vi "BalancePressure4.vi"(0 "FirgelliError":errorcluster, 1 "length":dbl=50.0 caption="Actuator Length (mm)", 2 "DesiredPressure":dbl=-0.08 min=-1.0 max=0.0 step=0.001, 3 "Position (mm)":dbl(slide)=25.0 min=0.0 max=50.0 step=0.2 scale=0.0..50.0 scale format="%.2f", 4 "ArduinoHandle":T2={"VISA resource"="", "Board Type"=enum."Uno", "Connection Type"=enum."USB / Serial", "Bytes Per Packet (15)"=15}, 5 "CurrentPressure":dbl, 6 "WRITE_HANDLE":u32 format="%04x", 7 "PressureOffset":dbl, 8 "READ_HANDLE":u32 format="%04x", 9 "Control Values":T1, 10 "Transducer (psi)":dbl(ring)=1.0 items=["+/- .18 psi"=1.0, "+/- .36 psi"=2.0, "+/- 1.08 psi"=3.0], 11 "Syringe (mL)":dbl(ring)=1.0 items=[".5 mL"=2.0, "1 mL"=1.0, "3 mL"=3.0]) -> (14 "FirgelliError Out":errorcluster, 15 "Control Values Out":T1, 16 "UpdateChart?":bool, 17 "Position (mm) Out":dbl(slide)=25.0 min=0.0 max=50.0 step=0.2 scale=0.0..50.0 scale format="%.2f", 18 "ArduinoError Out":errorcluster, 19 "Pressure (psi)":dbl)   [LabVIEW 2011]
uses:
  <vilib>/LabVIEW Interface for Arduino/Type Defs/Arduino Resource.ctl
  <vilib>/LabVIEW Interface for Arduino/Type Defs/Board Type.ctl
  orders/Firgelli motor/LAC_Software_V2/Firgelli Labview Example/Firgelli_LAC_LabVIEWsourceVer8_2/typeDefs/controlValues.ctl
  <vilib>/LabVIEW Interface for Arduino/LabVIEW Interface for Arduino.lvlib
panel:
  in  "Accuracy":dbl
  in  "P":dbl=4.0
  in  "stop 2":bool
  in  "stop":bool
  in  "D":dbl
  in  "I":dbl
  out "LastError":dbl
  out "Error":dbl
  out "LastPressure":dbl
  in  "ArduinoError":errorcluster
  in  "Analog Input Pin (0)":u8=1
  in  "Valve I/O Pin":u8=2
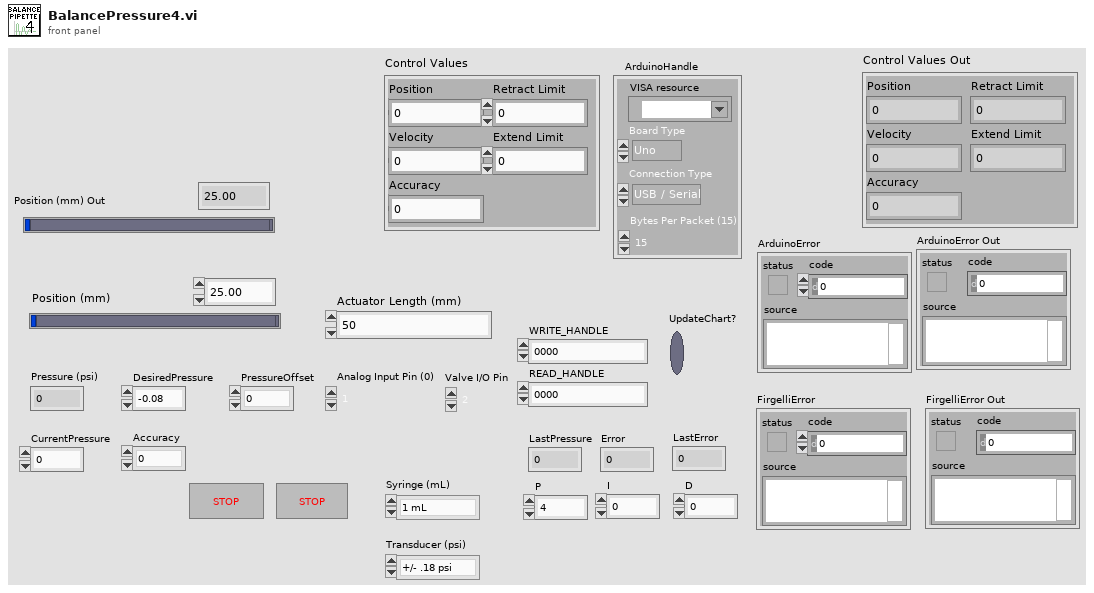
[diagram p1: front panel]
types:
  T1 = typedef "controlValues.ctl" = cluster{"Position":u16, "Velocity":u16, "Accuracy":u16, "Retract Limit":u16, "Extend Limit":u16}
  T2 = typedef "LabVIEW Interface for Arduino.lvlib/Arduino Resource.ctl" = cluster{"VISA resource":refnum<visa-resource-name>, "Board Type":T3, "Connection Type":enum8{"USB / Serial"}, "Bytes Per Packet (15)":u8}
  T3 = typedef "LabVIEW Interface for Arduino.lvlib/Board Type.ctl" = enum16{"Uno", "Dimuelanove w/Atmega 328", "Mega 2560"}
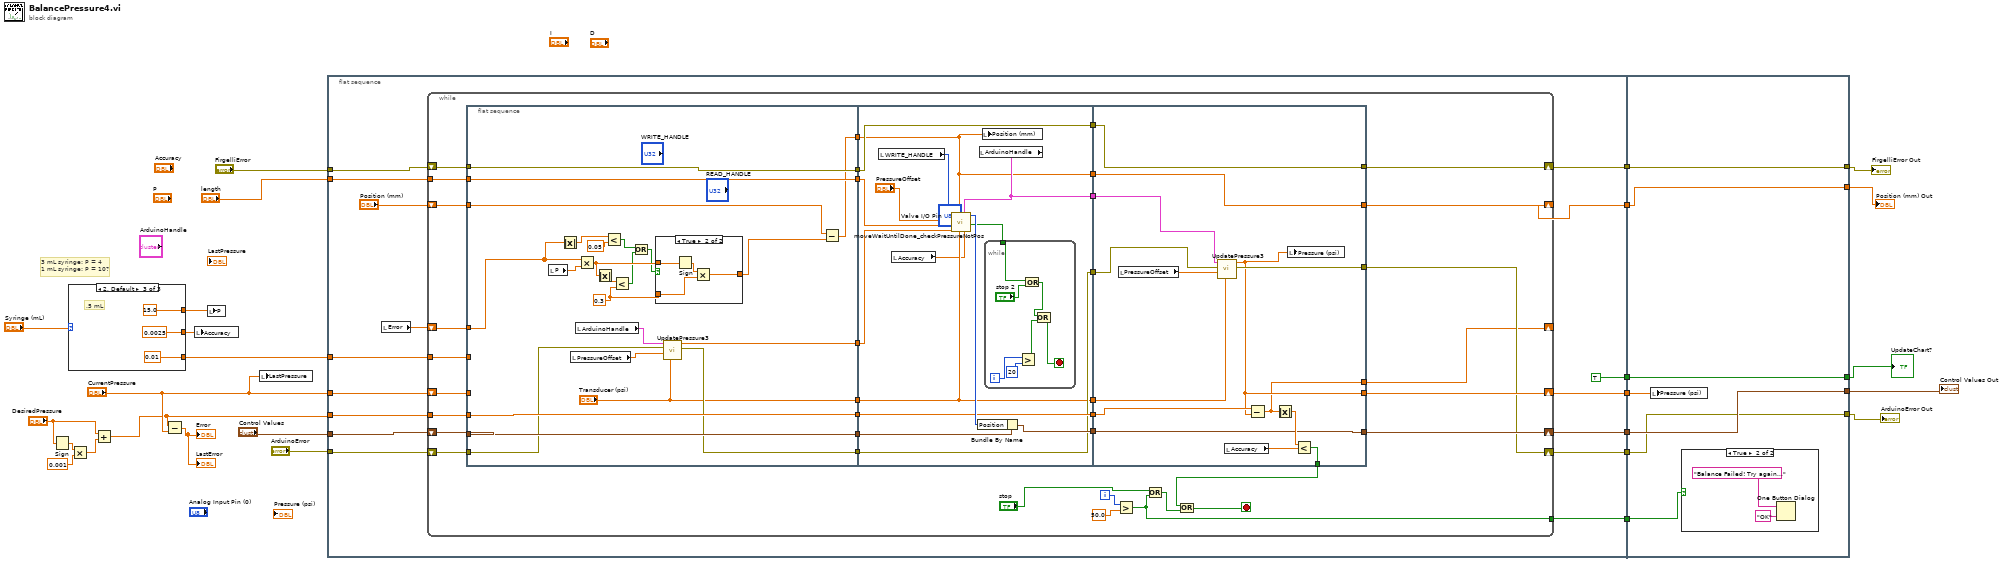
[diagram p0: block diagram]
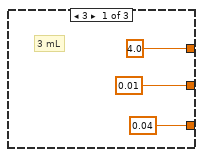
[diagram p2: hidden frame]
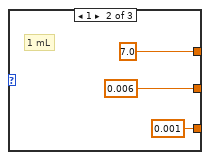
[diagram p3: hidden frame]
diagram:
  # "3 mL syringe: P = 4\n1 mL syringe: P = 10?"
  n1 = Sign(1:"DesiredPressure") -> (0:w3:dbl)
  n2 = case shown="2, Default" "Syringe (mL)" {
    tunnel: [4.0 ("P") 7.0 ("P") 15.0 ("P")] -> w8
    tunnel: [0.01 ("Accuracy") 0.006 ("Accuracy") 0.0025 ("Accuracy")] -> w7
    tunnel: [0.04 0.001 0.01] -> w6
    frame 3 {
      # "3 mL"
    }
    frame 1 {
      # "1 mL"
    }
    frame 2, Default {
      # ".5 mL"
    }
  }
  n3 = Multiply(x=w3, y=0.001) -> (x*y=w1:dbl)
  n4 = Add(x="DesiredPressure", y=w1) -> (x+y=w5:dbl)
  n5 = Subtract(x=w5, y="CurrentPressure") -> (x-y=→"Error" →"LastError":dbl)
  n6 = local write "Accuracy"(w7) -> ()
  n7 = local write "P"(w8) -> ()
  n8 = local write "LastPressure"("CurrentPressure") -> ()
  n9 = flat-sequence {
    tunnel: "CurrentPressure" -> [w52]
    tunnel: "FirgelliError" -> [w51]
    tunnel: "Control Values" -> [w50]
    tunnel: [w49] -> w27
    tunnel: [TRUE] -> w26
    tunnel: [w47] -> w25
    tunnel: [w46] -> w24
    tunnel: [w45] -> w23
    tunnel: [w38] -> w22
    tunnel: "ArduinoError" -> [w44]
    tunnel: w5 -> [w43]
    tunnel: [w41] -> w13
    tunnel: "length" -> [w39]
    tunnel: w6 -> [w37]
    tunnel: [w157] -> w17
    tunnel: [w158] -> w16
    tunnel: [w159] -> w15
    tunnel: [w160] -> w21
    tunnel: w27 -> [w156]
    tunnel: w26 -> [w160]
    tunnel: w25 -> [w159]
    tunnel: w24 -> [w158]
    tunnel: w23 -> [w157]
    tunnel: w22 -> [w155]
    tunnel: [w155] -> w14
    tunnel: w13 -> [w154]
    frame #0 {
      n10 = local read "Error"() -> (w40:dbl)
      n11 = while {
        shift-right: [w77] -> w49
        shift-left: w52 -> [w59]
        shift-right: [w60] -> w45
        shift-left: w51 -> [w85]
        tunnel: w39 -> [w83]
        shift-right: [w80] -> w47
        shift-left: w50 -> [w81]
        shift-right: [w71] -> w46
        shift-left: w44 -> [w78]
        tunnel: w43 -> [w88]
        shift-right: [w53] -> _
        shift-left: w40 -> [w75]
        tunnel: [w70] -> w41
        shift-right: [w72] -> w38
        shift-left: "Position (mm)" -> [w89]
        tunnel: w37 -> [w54]
        i -> [w74]
        stop <- w66 stop-if-true
        n12 = flat-sequence {
          tunnel: w89 -> [w108]
          tunnel: w88 -> [w109]
          tunnel: [w106] -> w87
          tunnel: [w112] -> w86
          tunnel: w85 -> [w112]
          tunnel: [w111] -> w84
          tunnel: w83 -> [w111]
          tunnel: [w110] -> w82
          tunnel: w81 -> [w110]
          tunnel: [w102] -> w79
          tunnel: w78 -> [w103]
          tunnel: [w109] -> w76
          tunnel: w75 -> [w94]
          tunnel: w59 -> [_]
          tunnel: [w104] -> w57
          tunnel: ["Transducer (psi)"] -> w55
          tunnel: w54 -> [_]
          tunnel: w87 -> [w120]
          tunnel: [w120] -> w65
          tunnel: w86 -> [w124]
          tunnel: w84 -> [w129]
          tunnel: w82 -> [w132]
          tunnel: [w131] -> w64
          tunnel: w79 -> [w126]
          tunnel: [w126] -> w63
          tunnel: w76 -> [w127]
          tunnel: [w127] -> w62
          tunnel: [w124] -> w61
          tunnel: [w122] -> w58
          tunnel: w57 -> [w121]
          tunnel: [w119] -> w56
          tunnel: w55 -> [w119]
          tunnel: w65 -> [w153]
          tunnel: w64 -> [w148]
          tunnel: w63 -> [w150]
          tunnel: w62 -> [w146]
          tunnel: [w147] -> w69
          tunnel: [w153] -> w72
          tunnel: [w148] -> w80
          tunnel: [w151] -> w71
          tunnel: [w145] -> w77
          tunnel: [w144] -> w53
          tunnel: w61 -> [w143]
          tunnel: [w143] -> w60
          tunnel: w58 -> [w142]
          tunnel: w56 -> [w140]
          frame #0 {
            w98 = 0.3 ("y")
            n13 = local read "P"() -> (w99:dbl)
            n14 = Absolute Value(x=w94) -> (abs(x)=w93:dbl)
            n15 = local read "PressureOffset"() -> (w101:dbl)
            n16 = local read "ArduinoHandle"() -> (w105:T2)
            n17 = Multiply(x=w94, y=w99) -> (x*y=w97:dbl)
            n18 = Absolute Value(x=w97) -> (abs(x)=w96:dbl)
            n19 = Less?(x=w93, y=0.05) -> (x < y?=w90:bool)
            n20 = Less?(x=w96, y=w98) -> (x < y?=w91:bool)
            n21 = Or(x=w90, y=w91) -> (x .or. y?=w95:bool)
            n22 = case shown="True" w95 {
              tunnel: w98 -> [_ w115]
              tunnel: w97 -> [w113 w117]
              tunnel: [w113 w114] -> w107
              frame False {
              }
              frame True {
                n23 = Sign(1:w117) -> (0:w116:dbl)
                n24 = Multiply(x=w116, y=w115) -> (x*y=w114:dbl)
              }
            }
            n25 = call "UpdatePressure3.vi"("Transducer (psi)"="Transducer (psi)", "PressureOffset"=w101, "Arduino error in"=w103, "ArduinoHandle"=w105) -> ("Arduino error out"=w102:errorcluster, "Pressure (psi)"=w104:dbl)  [unwired: 6 in]
            n26 = Subtract(x=w108, y=w107) -> (x-y=w106:dbl)
          }
          frame #1 {
            n27 = local read "WRITE_HANDLE"() -> (w130:u32)
            n28 = local read "Accuracy"() -> (w118:dbl)
            n29 = local read "ArduinoHandle"() -> (w122:T2)
            n30 = call "moveWaitUntilDone_checkPressureNotPos.vi"("Accuracy"=w118, "ArduinoHandle"=w122, "Transducer (psi)"=w119, "Position (mm)"=w120, "Pressure (psi)"=w121, "maxLength"=w129, "PressureOffset"="PressureOffset", "WRITE_HANDLE"=w130) -> ("moveDone?"=w125:bool, "regSetting"=w128:u16)  [unwired: 2 in]
            n31 = Bundle By Name(cluster=w132, "Position"=w128) -> (w131:T1)
            n32 = local write "Position (mm)"(w120) -> ()
            n33 = while {
              tunnel: w125 -> [w139]
              i -> [w136]
              stop <- w133 stop-if-true
              n34 = Greater?(x=w136, y=20) -> (0:w134:bool)
              n35 = Or(x=w139, y="stop 2") -> (x .or. y?=w137:bool)
              n36 = Or(x=w137, y=w134) -> (x .or. y?=w133:bool)
            }
          }
          frame #2 {
            n37 = local read "PressureOffset"() -> (w149:dbl)
            n38 = call "UpdatePressure3.vi"("Transducer (psi)"=w140, "PressureOffset"=w149, "Arduino error in"=w150, "ArduinoHandle"=w142) -> ("Arduino error out"=w151:errorcluster, "Pressure (psi)"=w145:dbl)  [unwired: 6 in]
            n39 = local read "Accuracy"() -> (w141:dbl)
            n40 = Subtract(x=w146, y=w145) -> (x-y=w144:dbl)
            n41 = Absolute Value(x=w144) -> (abs(x)=w152:dbl)
            n42 = local write "Pressure (psi)"(w145) -> ()
            n43 = Less?(x=w152, y=w141) -> (x < y?=w147:bool)
          }
        }
        n44 = Greater?(x=w74, y=50.0) -> (0:w70:bool)
        n45 = Or(x="stop", y=w70) -> (x .or. y?=w67:bool)
        n46 = Or(x=w69, y=w67) -> (x .or. y?=w66:bool)
      }
    }
    frame #1 {
      n47 = local write "Pressure (psi)"(w156) -> ()
      n48 = case shown="True" w154 {
        frame False {
        }
        frame True {
          n49 = One Button Dialog(message="Balance Failed! Try again...", button name ("OK")="OK") -> ()  [unwired: 1 out]
        }
      }
    }
  }
  "UpdateChart?" <- w21
  "ArduinoError Out" <- w16
  "FirgelliError Out" <- w17
  "Control Values Out" <- w15
  "Position (mm) Out" <- w14
